vi "Read Sequence Data.vi"(8 "error in":errorcluster, 9 "Array":T3(array[cluster]) {"Voltage" format="%.3g"; "Slope" format="%.3g"; "Current" format="%.3g"; "Width" format="%.3g"}, 10 "Sequence Number":dbl=1.0, 11 "VISA resource name":refnum<visa-resource-name>) -> (0 "error out":errorcluster, 1 "Array Out":T1(array[cluster]) {"Ext. List Voltage" format="%.3g"; "Ext. List Current" format="%.3g"; "Ext. List Time" format="%.3g"; "Ext. List Time 2" format="%.3g"}, 3 "VISA resource name out":refnum<visa-resource-name>, 5 "Actibve Steps":bool[](array[boolean]))   [LabVIEW 2022 SP3]
uses:
  <instrlib>/BK Precision 911X Series/BK Precision 911X Series.lvlib
panel:
  in  "new element/subarray":T2
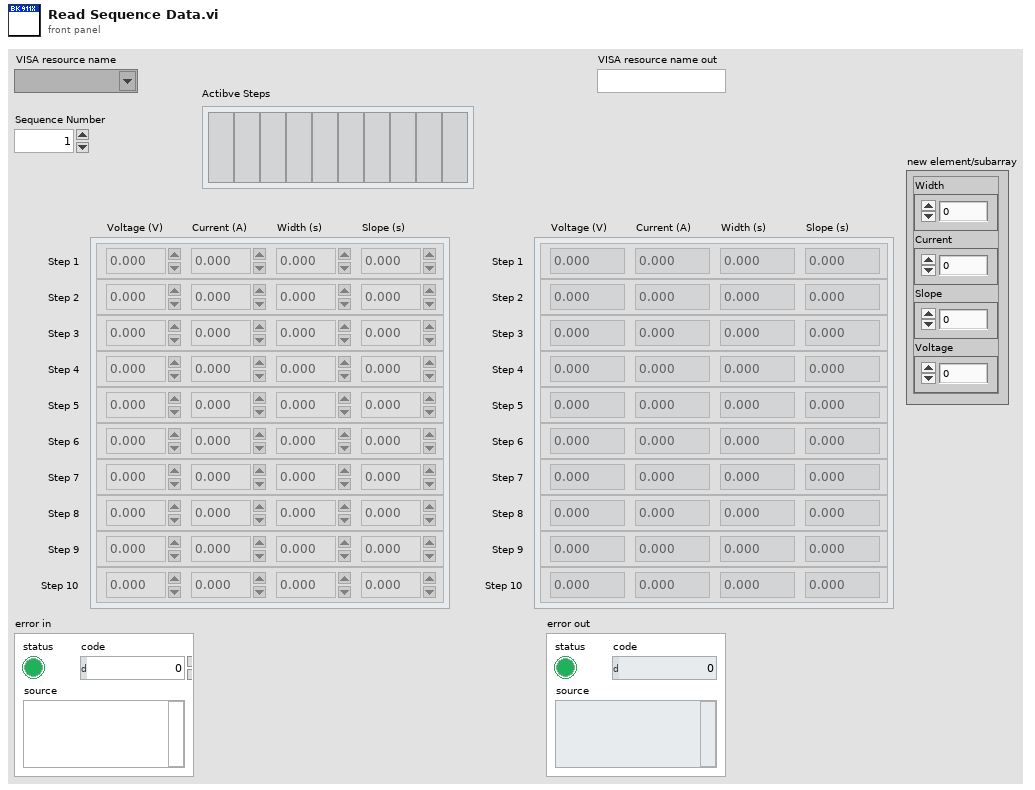
[diagram p1: front panel]
types:
  T1 = cluster{"Ext. List Time 2":dbl, "Ext. List Time":dbl, "Ext. List Current":dbl, "Ext. List Voltage ":dbl}[]
  T2 = cluster{"Width":dbl, "Current":dbl, "Slope":dbl, "Voltage ":dbl}
  T3 = cluster{"Width":dbl, "Current":dbl, "Slope":dbl, "Voltage":dbl}[]
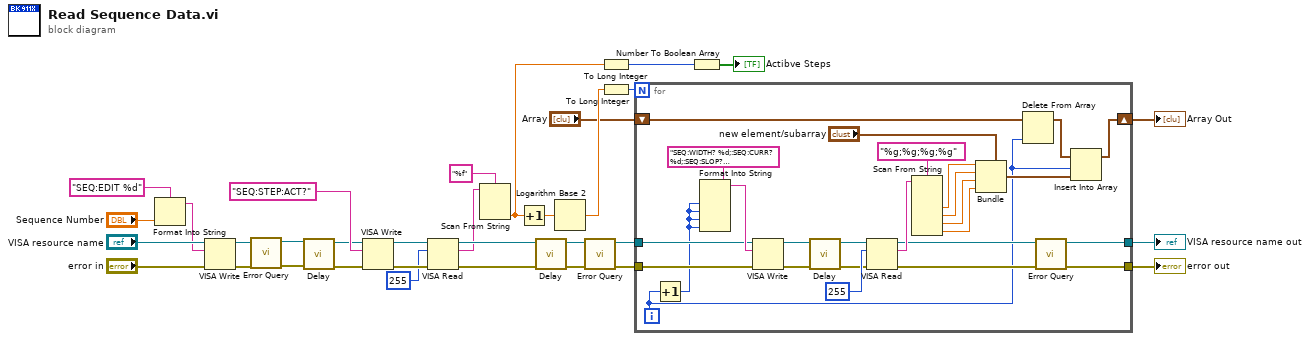
[diagram p0: block diagram]
diagram:
  n1 = Format Into String(format string="SEQ:EDIT %d" ("write buffer"), "Sequence Number") -> (resulting string=w30:string)  [unwired: 2 in, 1 out]
  n2 = VISA Write(VISA resource name="VISA resource name", write buffer=w30, error in (no error)="error in") -> (VISA resource name out=w13:refnum<visa-resource-name>, error out=w12:errorcluster)  [unwired: 1 out]
  n3 = call <instrlib>:"Error Query.vi"("error in (no error)"=w12, "VISA resource name"=w13) -> ("error out"=w10:errorcluster, "VISA resource name out"=w11:refnum<visa-resource-name>)  [unwired: 6 in, 2 out]
  n4 = call "Delay.vi"("error in (no error)"=w10, "VISA resource name"=w11) -> ("error out"=w14:errorcluster, "VISA resource name out"=w15:refnum<visa-resource-name>)  [unwired: 8 in]
  n5 = VISA Write(VISA resource name=w15, write buffer="SEQ:STEP:ACT?", error in (no error)=w14) -> (VISA resource name out=w27:refnum<visa-resource-name>, error out=w26:errorcluster)  [unwired: 1 out]
  n6 = VISA Read(VISA resource name=w27, byte count=u32 255, error in (no error)=w26) -> (VISA resource name out=w23:refnum<visa-resource-name>, read buffer=w9:string, error out=w22:errorcluster)  [unwired: 1 out]
  n7 = Scan From String(format string="%f", input string=w9) -> (output 1=w3:dbl)  [unwired: 3 in, 3 out]
  n8 = Increment(x=w3) -> (x+1=w5:dbl)
  n9 = call "Delay.vi"("error in (no error)"=w22, "VISA resource name"=w23) -> ("error out"=w20:errorcluster, "VISA resource name out"=w21:refnum<visa-resource-name>)  [unwired: 8 in]
  n10 = Logarithm Base 2(1:w5) -> (0:w8:dbl)
  n11 = call <instrlib>:"Error Query.vi"("error in (no error)"=w20, "VISA resource name"=w21) -> ("error out"=w18:errorcluster, "VISA resource name out"=w19:refnum<visa-resource-name>)  [unwired: 6 in, 2 out]
  n12 = To Long Integer(number=w3) -> (32bit integer=w4:i32)
  n13 = To Long Integer(number=w8) -> (32bit integer=w6:i32)
  n14 = for {
    N: w6 -> [_]
    tunnel: w19 -> [w58]
    tunnel: w18 -> [w57]
    tunnel: [w53] -> w17
    tunnel: [w52] -> w16
    shift-right: [w49] -> w1
    shift-left: "Array" -> [w36]
    i -> [w34]
    n15 = Increment(x=w34) -> (x+1=w51:i32)
    n16 = Format Into String(format string="SEQ:WIDTH? %d;:SEQ:CURR? %d;:SEQ:SLOP? %d;:SEQ:VOLT? %d", w51, w51, w51, w51) -> (resulting string=w59:string)  [unwired: 2 in, 1 out]
    n17 = VISA Write(VISA resource name=w58, write buffer=w59, error in (no error)=w57) -> (VISA resource name out=w42:refnum<visa-resource-name>, error out=w41:errorcluster)  [unwired: 1 out]
    n18 = call "Delay.vi"("error in (no error)"=w41, "VISA resource name"=w42) -> ("error out"=w39:errorcluster, "VISA resource name out"=w40:refnum<visa-resource-name>)  [unwired: 8 in]
    n19 = VISA Read(VISA resource name=w40, byte count=u32 255, error in (no error)=w39) -> (VISA resource name out=w38:refnum<visa-resource-name>, read buffer=w50:string, error out=w37:errorcluster)  [unwired: 1 out]
    n20 = Scan From String(format string="%g;%g;%g;%g", input string=w50) -> (output 1=w44:dbl, output 2=w45:dbl, output 3=w46:dbl, output 4=w47:dbl)  [unwired: 6 in, 3 out]
    n21 = Bundle(cluster="new element/subarray", "Width"=w44, "Current"=w45, "Slope"=w46, "Voltage"=w47) -> (w48:T2)
    n22 = Delete From Array(array=w36, index=w34) -> (array with subset deleted=w35:T3)  [unwired: 1 in, 1 out]
    n23 = call <instrlib>:"Error Query.vi"("error in (no error)"=w37, "VISA resource name"=w38) -> ("error out"=w53:errorcluster, "VISA resource name out"=w52:refnum<visa-resource-name>)  [unwired: 6 in, 2 out]
    n24 = Insert Into Array(array=w35, index=w34, new element=w48) -> (w49:T3)
  }
  "error out" <- w17
  "VISA resource name out" <- w16
  "Array Out" <- w1
  n25 = Number To Boolean Array(number=w4) -> (Boolean array=→"Actibve Steps":bool[])
